vi "State Change.vi"(8 "error in":errorcluster, 10 "Transition State":refnum<class "State Pattern.lvclass">, 11 "State Pattern in":refnum<class "State Pattern.lvclass">) -> (0 "error out":errorcluster, 3 "State Pattern out":refnum<class "State Pattern.lvclass">)   [LabVIEW 2021, in "State Pattern.lvclass"]
uses:
  State Pattern.lvclass
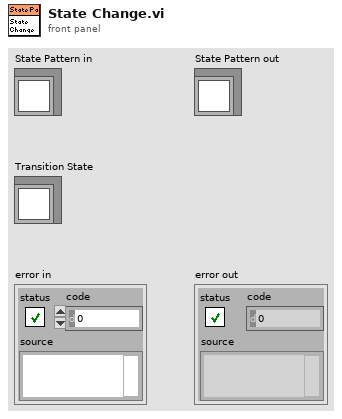
[diagram p1: front panel]
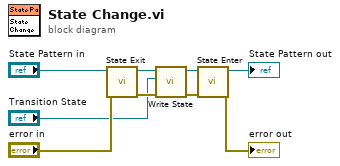
[diagram p0: block diagram]
diagram:
  n1 = call "State Exit.vi"("error in"="error in", "State Pattern in"="State Pattern in") -> ("error out"=w9:errorcluster, "State Pattern out"=w5:refnum<class "State Pattern.lvclass">)  [unwired: 8 in]
  n2 = call-dynamic "Write State.vi"("error in (no error)"=w9, "State"="Transition State", "State Pattern in"=w5) -> ("error out"=w8:errorcluster, "State Pattern out"=w4:refnum<class "State Pattern.lvclass">)  [unwired: 7 in]
  n3 = call "State Enter.vi"("error in"=w8, "State Pattern in"=w4) -> ("error out"=→"error out":errorcluster, "State Pattern out"=→"State Pattern out":refnum<class "State Pattern.lvclass">)  [unwired: 8 in]
